vi "ACT_Loop.vi"() -> ()   [LabVIEW 2020, in "Template_ACT.lvlib"]
uses:
  Template_ACT.lvlib
  Cluster_CMD_ACT_Data.ctl
  ENUM_ACT_State.ctl
  ENUM_ACT_Action.ctl
  Utility/Global_STOP.vi
  Global_CMD_ACT_Data In.vi
  Global_ACT_Data Out.vi
panel:
  out "Input DBL Data":T1
  out "Output DBL Data":dbl
  out "Cycle Time (S)":dbl format="%.3g"
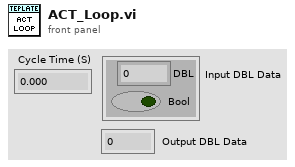
[diagram p1: front panel]
types:
  T1 = typedef "Template_ACT.lvlib/Cluster_CMD_ACT_Data.ctl" = cluster{"DBL":dbl, "Bool":bool}
  T2 = typedef "Template_ACT.lvlib/ENUM_ACT_State.ctl" = enum16{"Startup", "Idle", "Shutdown"}
  T3 = typedef "Template_ACT.lvlib/ENUM_ACT_Action.ctl" = enum16{"No Action", "Reset Time", "Reset All", "Action A", "Action B"}
  T4 = cluster{"Actuator Ref 0":cluster{i32}, "State":T2, "Previous State":T2, "Current Time":timestamp, "Previous Time":timestamp, "Start Time":timestamp, "Target Time (ms)":u32, "Cycle Time(S)":dbl, "ACT Input":T1, "ACT Output DBL":dbl}
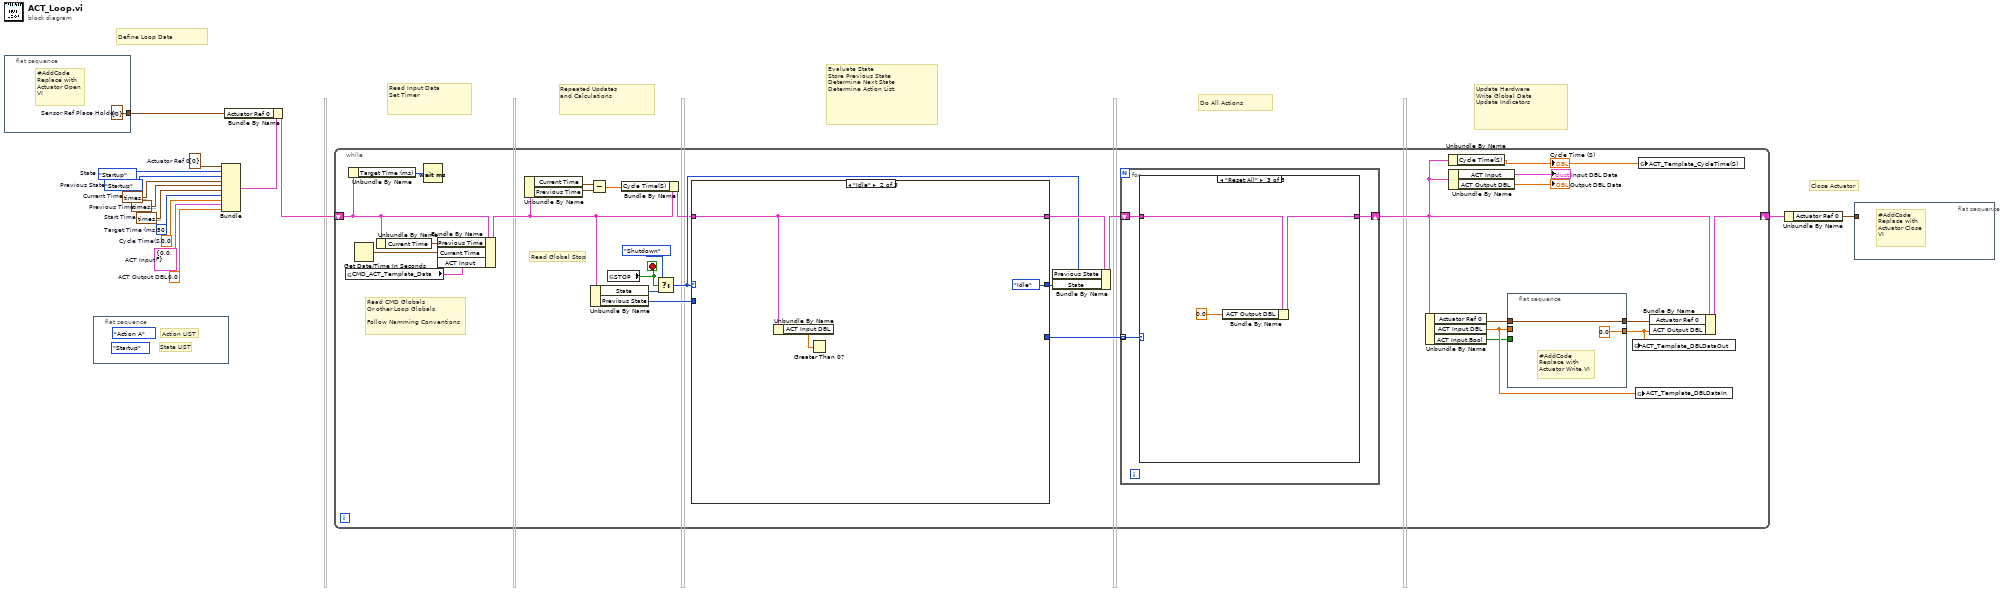
[diagram p0: block diagram]
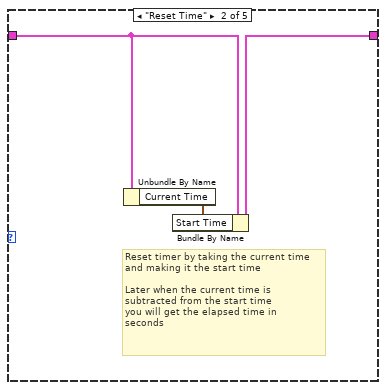
[diagram p3: hidden frame]
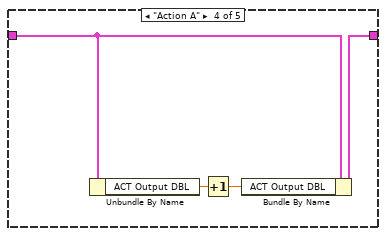
[diagram p4: hidden frame]
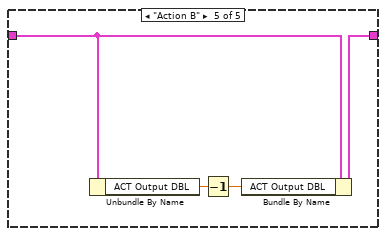
[diagram p5: hidden frame]
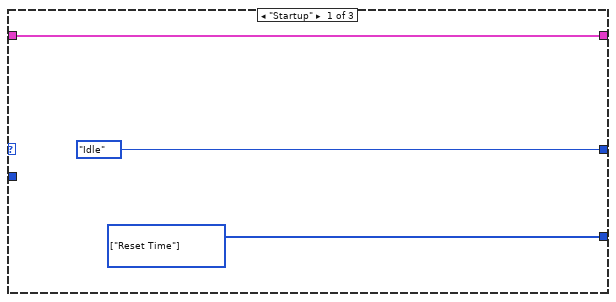
[diagram p6: hidden frame]
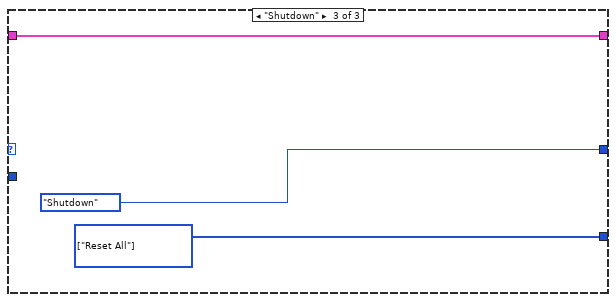
[diagram p7: hidden frame]
diagram:
  w4 = cluster{i32} {0}  # Actuator Ref 0
  w7 = 0.0  # Cycle Time(S)
  w8 = ENUM_ACT_State."Startup"  # Previous State
  w9 = timestamp(0 s since 1904-01-01)  # Previous Time
  w10 = u32 50  # Target Time (ms)
  w11 = 0.0  # ACT Output DBL
  w12 = T1 {"DBL"=0.0, "Bool"=FALSE}  # ACT Input
  w13 = timestamp(0 s since 1904-01-01)  # Start Time
  w14 = timestamp(0 s since 1904-01-01)  # Current Time
  w15 = ENUM_ACT_State."Startup"  # State
  # "Close Actuator"
  # "Define Loop Data"
  # "Repeated Updates\nand Calculations"
  # "Read Input Data\nSet Timer"
  # "Evaluate State\nStore Previous State\nDetermine Next State\nDetermine Action List"
  # "Do All Actions"
  # "Update Hardware\nWrite Global Data\nUpdate Indicators"
  n1 = flat-sequence {
    tunnel: [w16] -> w1
    frame #0 {
      w16 = cluster{i32} {0}  # Sensor Ref Place Holder
      # "#AddCode\nReplace with \nActuator Open\nVI"
    }
  }
  n2 = flat-sequence {
    frame #0 {
      (unwired) ENUM_ACT_State."Startup" ("State")
      (unwired) ENUM_ACT_Action."Action A" ("Action")
      # "State LIST"
      # "Action LIST"
    }
  }
  n3 = Bundle("Actuator Ref 0"=w4, "State"=w15, "Previous State"=w8, "Current Time"=w14, "Previous Time"=w9, "Start Time"=w13, "Target Time (ms)"=w10, "Cycle Time(S)"=w7, "ACT Input"=w12, "ACT Output DBL"=w11) -> (w3:T4)  [unwired: 1 in]
  n4 = Bundle By Name(cluster=w3, "Actuator Ref 0"=w1) -> (w2:T4)
  n5 = while {
    shift-right: [w21] -> w5
    shift-left: w2 -> [w36]
    stop <- w41 stop-if-true
    # "Read CMD Globals\nOr other Loop Globals\n\nFollow Namming Conventions"
    # "Read Global Stop"
    n6 = global read "Global_CMD_ACT_Data In.vi" "CMD_ACT_Template_Data"() -> (w25:T1)
    n7 = Unbundle By Name(w36) -> ("Target Time (ms)"=w38:u32)
    n8 = Get Date/Time In Seconds() -> (seconds since 1Jan1904=w45:timestamp)
    n9 = Unbundle By Name(w36) -> ("Current Time"=w37:timestamp)
    n10 = Wait (ms)(milliseconds to wait=w38) -> ()  [unwired: 1 out]
    n11 = Bundle By Name(cluster=w36, "Previous Time"=w37, "Current Time"=w45, "ACT Input"=w25) -> (w30:T4)
    n12 = Unbundle By Name(w30) -> ("Current Time"=w31:timestamp, "Previous Time"=w32:timestamp)
    n13 = Subtract(x=w31, y=w32) -> (x-y=w28:dbl)
    n14 = Unbundle By Name(w30) -> ("State"=w39:T2, "Previous State"=w35:T2)
    n15 = global read "Global_STOP.vi" "STOP"() -> (w41:bool)
    n16 = Bundle By Name(cluster=w30, "Cycle Time(S)"=w28) -> (w29:T4)
    n17 = Select(t=ENUM_ACT_State."Shutdown" ("State"), s=w41, f=w39) -> (s? t:f=w33:T2)
    n18 = case shown="\"Idle\"" w33 {
      tunnel: w29 -> [w68 w69 w74]
      tunnel: [w68 w69 w74] -> w43
      tunnel: [ENUM_ACT_State."Idle" ("State") ENUM_ACT_State."Idle" ("State") ENUM_ACT_State."Shutdown" ("State")] -> w42
      tunnel: [w67 _ w72] -> w27
      tunnel: w35 -> [_ _ _]
      frame "Startup" {
        w67 = T3[] [enum."Reset Time"] items=["No Action", "Reset Time", "Reset All", "Action A", "Action B"] ("Actions")
      }
      frame "Idle" {
        n19 = Unbundle By Name(w69) -> ("ACT Input.DBL"=w71:dbl)
        n20 = Greater Than 0?(x=w71) -> ()  [unwired: 1 out]
      }
      frame "Shutdown" {
        w72 = T3[] [enum."Reset All"] items=["No Action", "Reset Time", "Reset All", "Action A", "Action B"] ("Actions")
      }
    }
    n21 = Bundle By Name(cluster=w43, "Previous State"=w33, "State"=w42) -> (w44:T4)
    n22 = for {
      tunnel: w27 -> [w50] mode=indexing
      shift-right: [w49] -> w22
      shift-left: w44 -> [w48]
      n23 = case shown="\"Reset All\"" w50 {
        tunnel: w48 -> [w51 w54 w57 w60 w64]
        tunnel: [w51 w53 w56 w59 w63] -> w49
        frame "No Action" {
        }
        frame "Reset Time" {
          # "Reset timer by taking the current time\nand making it the start time\n\nLater when the current time is \nsubtracted from the start time\nyou will get the elapsed time in \nseconds"
          n24 = Unbundle By Name(w54) -> ("Current Time"=w52:timestamp)
          n25 = Bundle By Name(cluster=w54, "Start Time"=w52) -> (w53:T4)
        }
        frame "Reset All" {
          n26 = Bundle By Name(cluster=w57, "ACT Output DBL"=0.0 ("FG Write Value")) -> (w56:T4)
        }
        frame "Action A" {
          n27 = Unbundle By Name(w60) -> ("ACT Output DBL"=w61:dbl)
          n28 = Increment(x=w61) -> (x+1=w58:dbl)
          n29 = Bundle By Name(cluster=w60, "ACT Output DBL"=w58) -> (w59:T4)
        }
        frame "Action B" {
          n30 = Unbundle By Name(w64) -> ("ACT Output DBL"=w65:dbl)
          n31 = Decrement(x=w65) -> (x-1=w62:dbl)
          n32 = Bundle By Name(cluster=w64, "ACT Output DBL"=w62) -> (w63:T4)
        }
      }
    }
    n33 = Unbundle By Name(w22) -> ("Actuator Ref 0"=w24:cluster{i32}, "ACT Input.DBL"=w19:dbl, "ACT Input.Bool"=w17:bool)
    n34 = Unbundle By Name(w22) -> ("Cycle Time(S)"=w20:dbl)
    "Cycle Time (S)" <- w20
    n35 = Unbundle By Name(w22) -> ("ACT Input"=→"Input DBL Data":T1, "ACT Output DBL"=→"Output DBL Data":dbl)
    n36 = flat-sequence {
      tunnel: w24 -> [w47]
      tunnel: [w47] -> w23
      tunnel: w19 -> [_]
      tunnel: [0.0 ("ACT_Template_DBLDataOut")] -> w18
      tunnel: w17 -> [_]
      frame #0 {
        # "#AddCode\nReplace with\nActuator Write VI"
      }
    }
    n37 = global write "Global_ACT_Data Out.vi" "ACT_Template_DBLDataOut"(w18) -> ()
    n38 = global write "Global_ACT_Data Out.vi" "ACT_Template_DBLDataIn"(w19) -> ()
    n39 = global write "Global_ACT_Data Out.vi" "ACT_Template_CycleTime(S)"(w20) -> ()
    n40 = Bundle By Name(cluster=w22, "Actuator Ref 0"=w23, "ACT Output DBL"=w18) -> (w21:T4)
  }
  n41 = Unbundle By Name(w5) -> ("Actuator Ref 0"=w6:cluster{i32})
  n42 = flat-sequence {
    tunnel: w6 -> [_]
    frame #0 {
      # "#AddCode\nReplace with \nActuator Close\nVI"
    }
  }
